vi "encoder2mps.vi"(6 "Gear":enum16{"7", "6", "5", "4", "3", "2", "1"}(ring), 11 "encoderSpeed":dbl) -> (3 "realVelocity":dbl)   [LabVIEW 2016]
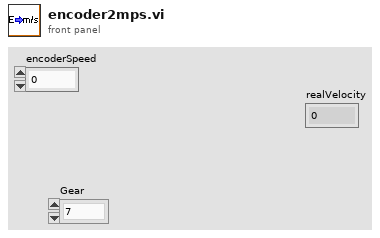
[diagram p1: front panel]
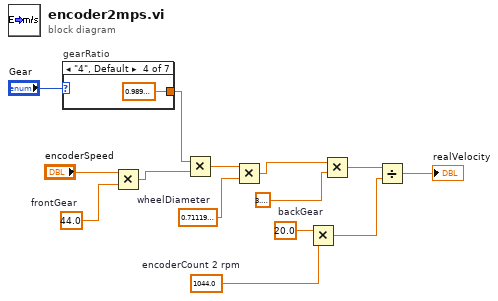
[diagram p0: block diagram]
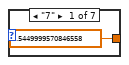
[diagram p2: hidden frame]
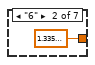
[diagram p3: hidden frame]
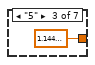
[diagram p4: hidden frame]
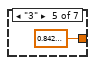
[diagram p5: hidden frame]
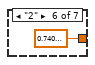
[diagram p6: hidden frame]
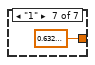
[diagram p7: hidden frame]
diagram:
  w3 = 1044.0  # encoderCount 2 rpm
  w4 = 20.0  # backGear
  w8 = 0.7111999988555908  # wheelDiameter
  w12 = 44.0  # frontGear
  n1 = case "gearRatio" shown="\"4\", Default" "Gear" {
    tunnel: [1.5449999570846558 1.3350000381469727 1.1449999809265137 0.9890000224113464 0.8429999947547913 0.7409999966621399 0.6320000290870667] -> w10
    frame "7" {
    }
    frame "6" {
    }
    frame "5" {
    }
    frame "4", Default {
    }
    frame "3" {
    }
    frame "2" {
    }
    frame "1" {
    }
  }
  n2 = Multiply(x="encoderSpeed", y=w12) -> (x*y=w11:dbl)
  n3 = Multiply(x=w10, y=w11) -> (x*y=w9:dbl)
  n4 = Multiply(x=w9, y=w8) -> (x*y=w1:dbl)
  n5 = Multiply(x=w4, y=w3) -> (x*y=w5:dbl)
  n6 = Multiply(x=w1, y=3.141592653589793) -> (x*y=w6:dbl)
  n7 = Divide(x=w6, y=w5) -> (x/y=→"realVelocity":dbl)
